vi "OVLD check.vi"(8 "error in (no error)":errorcluster, 10 "Measurement (in)":string, 11 "VISA resource name":refnum<visa-resource-name>) -> (0 "error out":errorcluster, 2 "Measurement (out)":dbl, 3 "VISA resource name out":refnum<visa-resource-name>)   [LabVIEW 2020, in "PICOTEST M351XA Series.lvlib"]
doc: "The OVLD check verify the measurement (in) by M351X function.\n\nfunction \"DIODE\" :\ngreater then 1.2\n\nthe other function :\nmeasurement (in) value equal to 9.9E+37."
uses:
  PICOTEST M351XA Series.lvlib
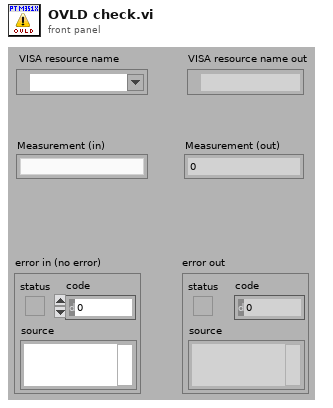
[diagram p1: front panel]
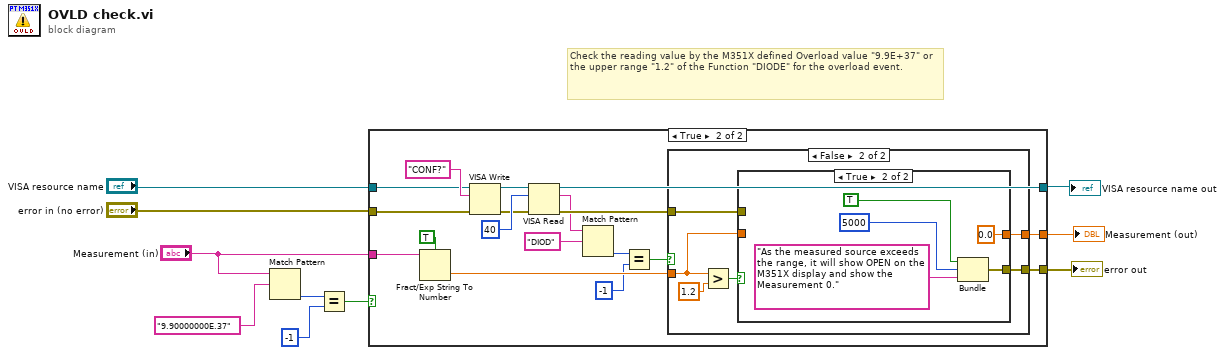
[diagram p0: block diagram]
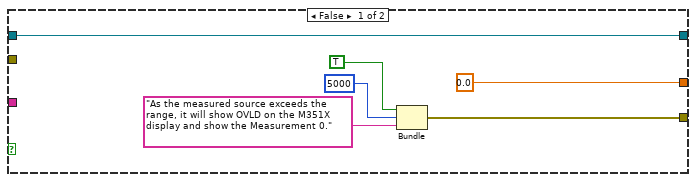
[diagram p2: hidden frame]
diagram:
  # "Check the reading value by the M351X defined Overload value \"9.9E+37\" or \nthe upper range \"1.2\" of the Function \"DIODE\" for the overload event."
  n1 = Match Pattern(string="Measurement (in)", regular expression="9.90000000E.37") -> (offset past match=w9:i32)  [unwired: 1 in, 3 out]
  n2 = Equal?(x=w9, y=-1) -> (x = y?=w5:bool)
  n3 = case shown="True" w5 {
    tunnel: [0.0 w28] -> w1
    tunnel: "error in (no error)" -> [_ w26]
    tunnel: "VISA resource name" -> [w15 w30]
    tunnel: [w11 w27] -> w7
    tunnel: [w15 w24] -> w6
    tunnel: "Measurement (in)" -> [_ w18]
    frame False {
      n4 = Bundle(TRUE, 5000, "As the measured source exceeds the range, it will show OVLD on the M351X display and show the Measurement 0.") -> (w11:errorcluster)  [unwired: 1 in]
    }
    frame True {
      n5 = Fract/Exp String To Number(use system decimal point (T)=TRUE, string=w18) -> (number=w29:dbl)  [unwired: 2 in, 1 out]
      n6 = VISA Write(VISA resource name=w30, write buffer="CONF?", error in (no error)=w26) -> (VISA resource name out=w32:refnum<visa-resource-name>, error out=w31:errorcluster)  [unwired: 1 out]
      n7 = VISA Read(VISA resource name=w32, byte count=u32 40, error in (no error)=w31) -> (VISA resource name out=w24:refnum<visa-resource-name>, read buffer=w23:string, error out=w25:errorcluster)  [unwired: 1 out]
      n8 = Match Pattern(string=w23, regular expression="DIOD") -> (offset past match=w21:i32)  [unwired: 1 in, 3 out]
      n9 = Equal?(x=w21, y=-1) -> (x = y?=w19:bool)
      n10 = case shown="False" w19 {
        tunnel: w29 -> [w36 w38]
        tunnel: [w36 w40] -> w28
        tunnel: [w35 w39] -> w27
        tunnel: w25 -> [w35 w37]
        frame True {
        }
        frame False {
          n11 = Greater?(x=w38, y=1.2) -> (0:w41:bool)
          n12 = case shown="True" w41 {
            tunnel: [w44 0.0] -> w40
            tunnel: [w43 w45] -> w39
            tunnel: w38 -> [w44 _]
            tunnel: w37 -> [w43 _]
            frame False {
            }
            frame True {
              n13 = Bundle(TRUE, 5000, "As the measured source exceeds the range, it will show OPEN on the M351X display and show the Measurement 0.") -> (w45:errorcluster)  [unwired: 1 in]
            }
          }
        }
      }
    }
  }
  "VISA resource name out" <- w6
  "error out" <- w7
  "Measurement (out)" <- w1
